vi "Close_Instr.vi"(8 "error in (no error)":errorcluster caption="entrée d'erreur (pas d'erreur)", 11 "Class Instrument Multimeter en entrée":refnum<class "Class Instrument Balance.lvclass">) -> (0 "error out":errorcluster caption="sortie d'erreur", 3 "Class Instrument Multimeter en sortie":refnum<class "Class Instrument Balance.lvclass">)   [LabVIEW 2020, in "Library Instrument & Equipement.lvlib" / "Library Instruments.lvlib" / "Class Instrument Balance.lvclass"]
uses:
  Class Instrument Balance.lvclass
  Class Instrument Balance.lvclass/Class Instrument Balance.ctl
  Balance/Balance (Default)/Class Balance (Default).lvclass
  Instrument (Default)/Class Instrument (Default).lvclass
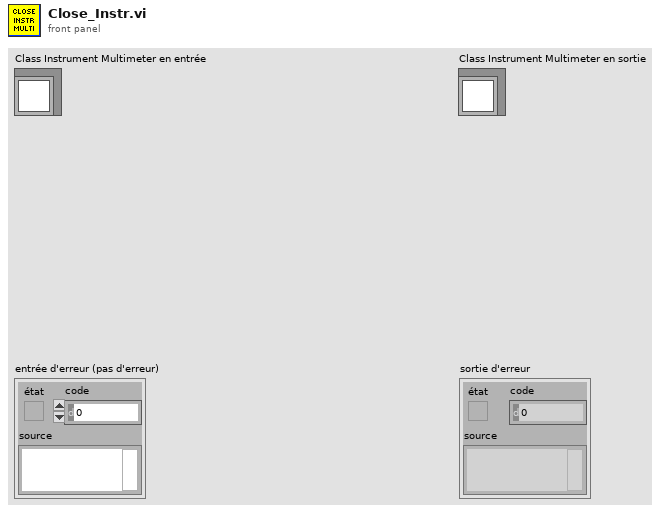
[diagram p1: front panel]
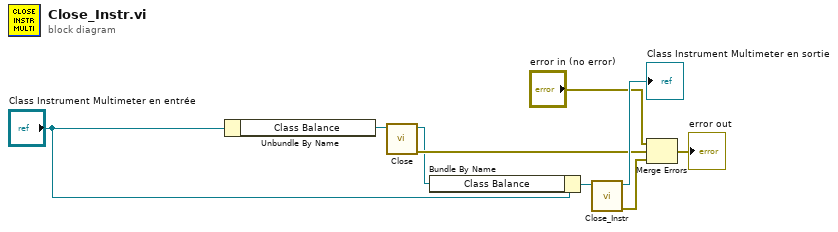
[diagram p0: block diagram]
diagram:
  n1 = Unbundle By Name("Class Instrument Multimeter en entrée") -> ("Class Balance"=w3:refnum<class "Class Balance (Default).lvclass">)
  n2 = call-dynamic "Close.vi"("Class Balance (Default) en entrée"=w3) -> ("error out"=w2:errorcluster, "Class Balance (Default) en sortie"=w1:refnum<class "Class Balance (Default).lvclass">)  [unwired: 9 in]
  n3 = Bundle By Name(cluster="Class Instrument Multimeter en entrée", "Class Balance"=w1) -> (w7:refnum<class "Class Instrument Balance.lvclass">)
  n4 = call-parent "Close_Instr.vi"("Class Instrument (Default) en entrée"=w7) -> ("error out"=w5:errorcluster, "Class Instrument (Default) en sortie"=→"Class Instrument Multimeter en sortie":refnum<class "Class Instrument Balance.lvclass">)  [unwired: 9 in]
  n5 = Merge Errors("error in (no error)", w2, w5) -> (→"error out":errorcluster)
